vi "Logger.vi"(8 "Time Between Loops":i64=25, 10 "Data":dbl[](array[numeric]), 11 "Header Line":string="Time\tDelta_Time\tSlider\n") -> ()   [LabVIEW 2018]
uses:
  <vilib>/Platform/TimedLoop/XDataNode/timing_clust.ctl
  <vilib>/Platform/TimedLoop/XDataNode/nitl_modes.ctl
  <vilib>/Platform/TimedLoop/XDataNode/wakeup.ctl
  <vilib>/Platform/TimedLoop/XDataNode/XDataNode.xnode
  <vilib>/Platform/TimedLoop/XDataNode/XDNodeRunTimeDep.lvlib
panel:
  out "Path":path
  out "Number of Log Entries":i32
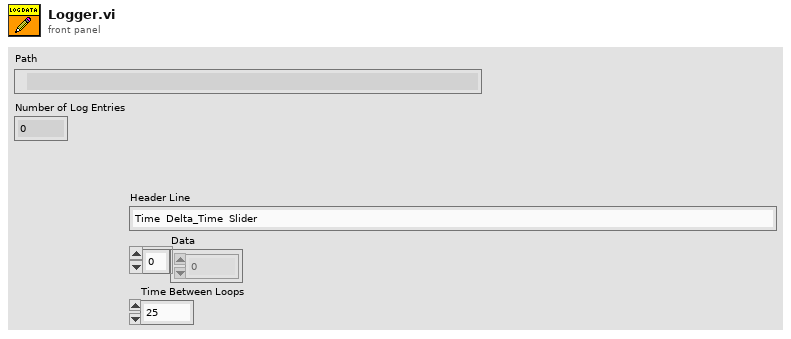
[diagram p1: front panel]
types:
  T1 = enum16{"open", "replace", "create", "open or create", "replace or create", "replace or create with confirmation"}
  T2 = typedef "NetComm_MatchType.ctl" = enum32{"None", "Practice", "Qualification", "Elimination"}
  T3 = typedef "WPI_DriverStationPositionInfo.ctl" = enum16{"1", "2", "3"}
  T4 = typedef "WPI_DriverStationAllianceInfo.ctl" = enum16{"Red", "Blue", "Invalid"}
  T5 = typedef "XDNodeRunTimeDep.lvlib/timing_clust.ctl" = cluster{"Expected End [f-1]":u64, "Actual End [f-1]":u64, "Finished Late? [f-1]":bool, "Expected End [i-1]":u64, "Actual End [i-1]":u64, "Finished Late? [i-1]":bool, "Expected Start [i]":u64, "Actual Start [i]":u64, "Expected Start [f]":u64, "Actual Start [f]":u64, "Source Name":string, "Structure Name":string, "Period":i64, "Deadline":i64, "Offset":i64, "Start":i64, "Priority":i32, "Timeout":i32, "Mode":T6, "Wakeup Reason":T7, "Error":errorcluster, "Source Type":string, "Secondary Source Type":string, "Global End Time":u64, "Global Start Time":u64, "Frame Duration":u64, "Iteration Duration":u64, "Assigned CPU":i32, "I/O Scan Engine Mode":u32}
  T6 = typedef "XDNodeRunTimeDep.lvlib/nitl_modes.ctl" = enum32{"No Change", "Process missed periods, maintain original phase", "Discard missed periods, maintain original phase", "Process missed periods, ignore original phase", "Discard missed periods, ignore original phase"}
  T7 = typedef "XDNodeRunTimeDep.lvlib/wakeup.ctl" = enum32{"Normal", "Aborted", "Asynchronous wakeup", "Timing source error", "Timed loop error", "Timeout"}
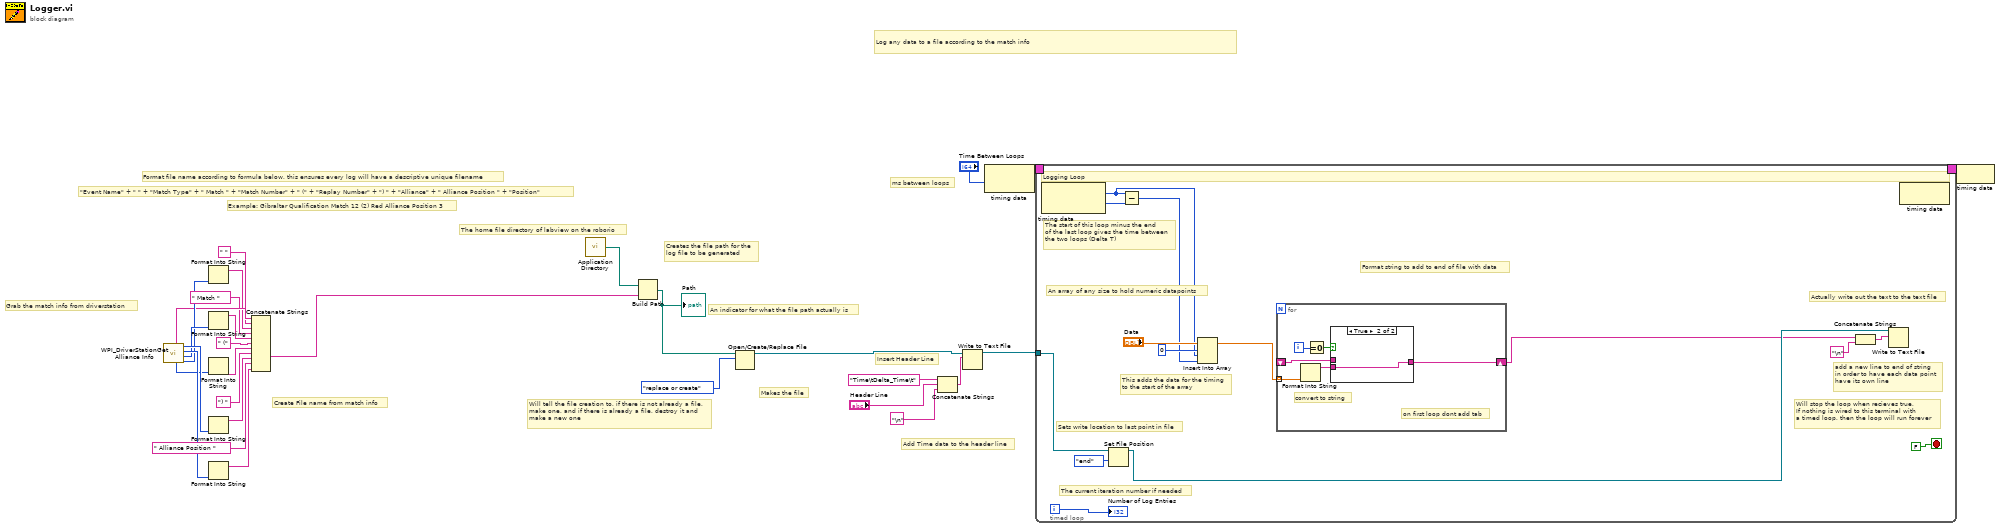
[diagram p0: block diagram]
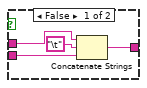
[diagram p2: hidden frame]
diagram:
  # "Log any data to a file according to the match info"
  # "Add Time data to the header line"
  # "Insert Header Line"
  # "Create File name from match info"
  # "Grab the match info from driverstation"
  # "Format file name according to formula below, this ensures every log will have a descriptive unique filename"
  # "Example: Gibraltar Qualification Match 12 (2) Red Alliance Position 3"
  # "\"Event Name\" + \" \" + \"Match Type\" + \" Match \" + \"Match Number\" + \" (\" + \"Replay Number\" + \") \" + \"Alliance\" + \" Alliance Position \" + \"Position\""
  # "Makes the file"
  # "Will tell the file creation to, if there is not already a file,\nmake one, and if there is already a file, destroy it and\nmake a new one"
  # "An indicator for what the file path actually is"
  # "Creates the file path for the\nlog file to be generated"
  # "The home file directory of labview on the roborio"
  # "ms between loops"
  n1 = call <vilib>:"WPI_DriverStationGet Alliance Info.vi"() -> ("Match Type"=w20:T2, "Match Number"=w21:u16, "Position"=w22:T3, "Alliance"=w23:T4, "Replay Number"=w19:u16, "Event Name"=w18:string)  [unwired: 6 in]
  n2 = Format Into String(w20) -> (resulting string=w16:string)  [unwired: 3 in, 1 out]
  n3 = Format Into String(w21) -> (resulting string=w14:string)  [unwired: 3 in, 1 out]
  n4 = Format Into String(w19) -> (resulting string=w12:string)  [unwired: 3 in, 1 out]
  n5 = Format Into String(w23) -> (resulting string=w10:string)  [unwired: 3 in, 1 out]
  n6 = Format Into String(w22) -> (resulting string=w8:string)  [unwired: 3 in, 1 out]
  n7 = Concatenate Strings(w18, " " ("string"), w16, " Match " ("string"), w14, " (" ("string"), w12, ") " ("string"), w10, " Alliance Position " ("string"), w8) -> (w7:string)
  n8 = call <vilib>:"Application Directory.vi"() -> ("Application Directory"=w25:path)
  n9 = Build Path(base path=w25, name or relative path=w7) -> (appended path=w24:path)
  "Path" <- w24
  n10 = Open/Create/Replace File(file path (use dialog)=w24, operation (0:open)=T1."replace or create") -> (refnum out=w6:refnum<file>)  [unwired: 4 in, 2 out]
  n11 = Concatenate Strings("Time\tDelta_Time\t", "Header Line", "\n") -> (w2:string)
  n12 = Write to Text File(file (use dialog)=w6, text=w2) -> (refnum out=w5:refnum<file>)  [unwired: 2 in, 2 out]
  n13 = node-c288("Time Between Loops") -> (w29:T5)
  n14 = timed-loop {
    timing: w29 -> [_]
    timing-out: [_] -> w28
    tunnel: w5 -> [w41]
    i -> [w37]
    stop <- FALSE stop-if-true
    # "An array of any size to hold numeric datapoints"
    # "This adds the data for the timing\nto the start of the array"
    # "Format string to add to end of file with data"
    # "The current iteration number if needed"
    # "Will stop the loop when recieves true,\nIf nothing is wired to this terminal with\na timed loop, then the loop will run forever"
    # "Actually write out the text to the text file"
    # "add a new line to end of string\nin order to have each data point\nhave its own line"
    # "The start of this loop minus the end\nof the last loop gives the time between\nthe two loops (Delta T)"
    # "Sets write location to last point in file"
    # "Logging Loop"
    n15 = node-c288() -> (w32:i64, w38:i64)  [unwired: 1 in]
    n16 = Set File Position(refnum=w41, from (0:start)=enum16{"start", "end", "current"}."end") -> (refnum out=w42:refnum<file>)  [unwired: 2 in, 1 out]
    n17 = Subtract(x=w32, y=w38) -> (x-y=w31:i64)
    n18 = Insert Into Array(array="Data", index=0, new element #1=w32, new element #2=w31) -> (w30:dbl[])
    n19 = for {
      tunnel: w30 -> [w49] mode=indexing
      shift-right: [w45] -> w35
      shift-left: _ -> [w44]
      i -> [w48]
      # "on first loop dont add tab"
      # "convert to string"
      n20 = Format Into String(w49) -> (resulting string=w46:string)  [unwired: 3 in, 1 out]
      n21 = Equal To 0?(x=w48) -> (x = 0?=w47:bool)
      n22 = case shown="True" w47 {
        tunnel: w46 -> [w51 w54]
        tunnel: [w50 w54] -> w45
        tunnel: w44 -> [w53 _]
        frame False {
          n23 = Concatenate Strings(w53, "\t", w51) -> (w50:string)
        }
        frame True {
        }
      }
    }
    n24 = Concatenate Strings(w35, "\n" ("string")) -> (w40:string)
    n25 = Write to Text File(file (use dialog)=w42, text=w40) -> ()  [unwired: 2 in, 3 out]
    n26 = node-c288() -> ()  [unwired: 1 in, 1 out]
    "Number of Log Entries" <- w37
  }
  n27 = node-c288(w28) -> ()
